vi "SIMPID(v.2).vi"(3 "Range":dbl=10.0, 5 "upper limit":dbl=1.0, 7 "lower limit":dbl=0.4, 9 "Current Point":dbl(knob) scale=0.0..200.0, 10 "Set Point":dbl(knob) scale=0.0..200.0, 11 "Gain Max":dbl=1.0) -> (0 "On Target":bool, 1 "result":dbl)   [LabVIEW 2011]
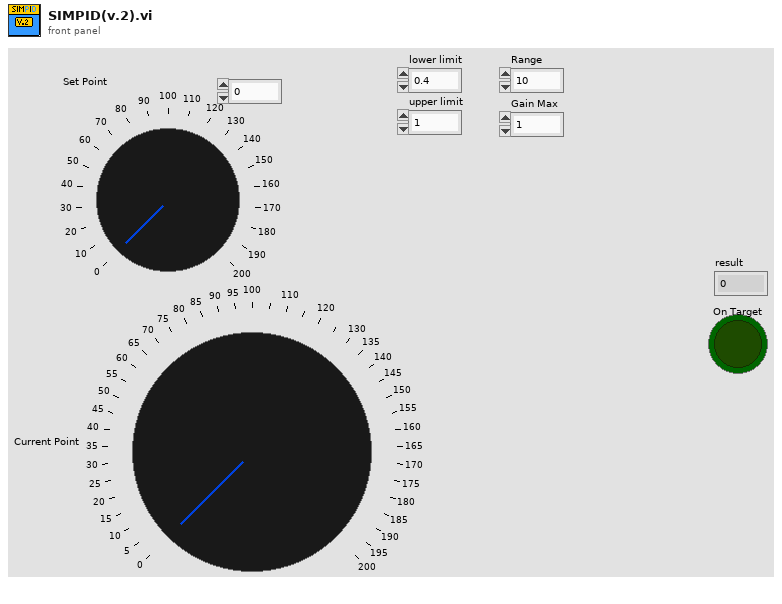
[diagram p1: front panel]
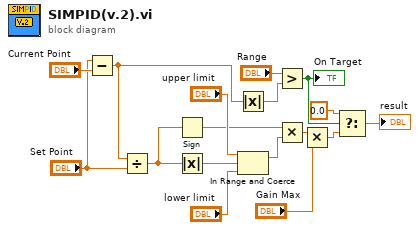
[diagram p0: block diagram]
diagram:
  n1 = Subtract(x="Set Point", y="Current Point") -> (x-y=w4:dbl)
  n2 = Divide(x=w4, y="Set Point") -> (x/y=w14:dbl)
  n3 = Sign(1:w14) -> (0:w11:dbl)
  n4 = Absolute Value(x=w14) -> (abs(x)=w15:dbl)
  n5 = Absolute Value(x=w4) -> (abs(x)=w9:dbl)
  n6 = In Range and Coerce(upper limit="upper limit", x=w15, lower limit="lower limit") -> (coerced(x)=w10:dbl)  [unwired: 1 out]
  n7 = Greater?(x="Range", y=w9) -> (0:w8:bool)
  "On Target" <- w8
  n8 = Multiply(x=w11, y=w10) -> (x*y=w3:dbl)
  n9 = Multiply(x=w3, y="Gain Max") -> (x*y=w2:dbl)
  n10 = Select(t=0.0, s=w8, f=w2) -> (s? t:f=→"result":dbl)
